vi "MALT132 Get Several.vi"(8 "error in":errorcluster, 9 "port":i32, 10 "Address":i32, 11 "MALT CardType":T1=enum."MALT132") -> (0 "error out":errorcluster, 3 "Status":u8[](array[numeric]) format="%02x")   [LabVIEW 2018]
uses:
  Types/MALT CardTypes.ctl
panel:
  out "Response":string
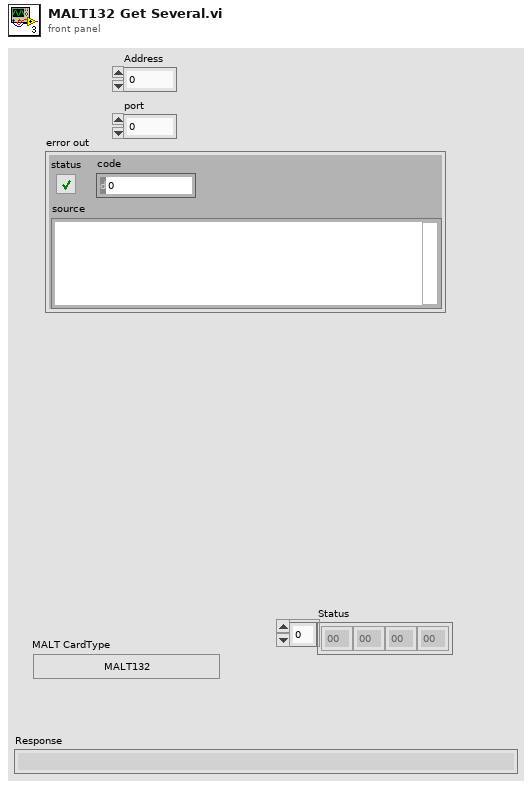
[diagram p1: front panel]
types:
  T1 = typedef "MALT CardTypes.ctl" = enum32{"-", "YAV90832", "YAV904X8", "MALT132", "YAV91616", "YAV90PIN", "YAV90096", "YAV90HVT", "YAV90CLR", "YAV90128", "YAV90PNE", "YAVCANCON", "YAV91775", "YAV90XXX", "YAV90MMU", "H730050", "H710060", "H710061", "YAV90304", "MMI", "YAV90060", "YAV90MUX", "YAV90059", "Not Defined"}
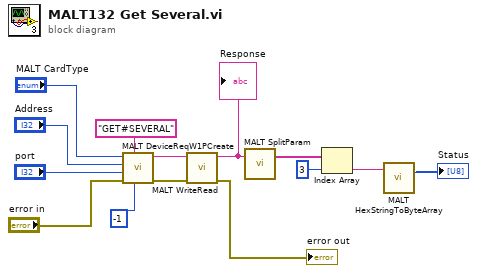
[diagram p0: block diagram]
diagram:
  n1 = call "MALT DeviceReqW1PCreate.vi"(6:-1 ("Block"), "Cmd"="GET#SEVERAL" ("cmd"), "error in"="error in", "Param1"="port", "Address"="Address", "CardType"="MALT CardType") -> ("error out"=w6:errorcluster, "Request"=w10:string)  [unwired: 4 in]
  n2 = call "MALT WriteRead.vi"("error in"=w6, "Request"=w10) -> ("error out"=→"error out":errorcluster, "Response"=w14:string)  [unwired: 8 in]
  "Response" <- w14
  n3 = call "MALT SplitParam.vi"("Line"=w14) -> ("Items"=w12:string[])  [unwired: 2 in]
  n4 = Index Array(array=w12, index=3) -> (element=w2:string)
  n5 = call "MALT HexStringToByteArray.vi"("String in"=w2) -> ("Bytes out"=→"Status":u8[])  [unwired: 2 in]
